vi "글로벌 1.vi"() -> ()   [LabVIEW 2017, in "Serial Communcation Devices Custom Device.lvlib"]
uses:
  Serial Communcation Devices Custom Device.lvlib
panel:
  in  "Channel Setting GUID":string
  out "GUID (Default Channel)":string="03D3BB99-1485-13A6-561D1F898F032919"
  in  "Flow Control":string
  in  "Stop Bits":string
  in  "Parity":string
  in  "Data Bits":string
  in  "Baud Rate":string
  in  "VISA Resource Name":string
  in  "Timeout(ms)":string
  in  "Enable Termination Char":string
  in  "Device GUID":string
  # "43b76903-71cc-4e2b-b034-344d1b7f9646"
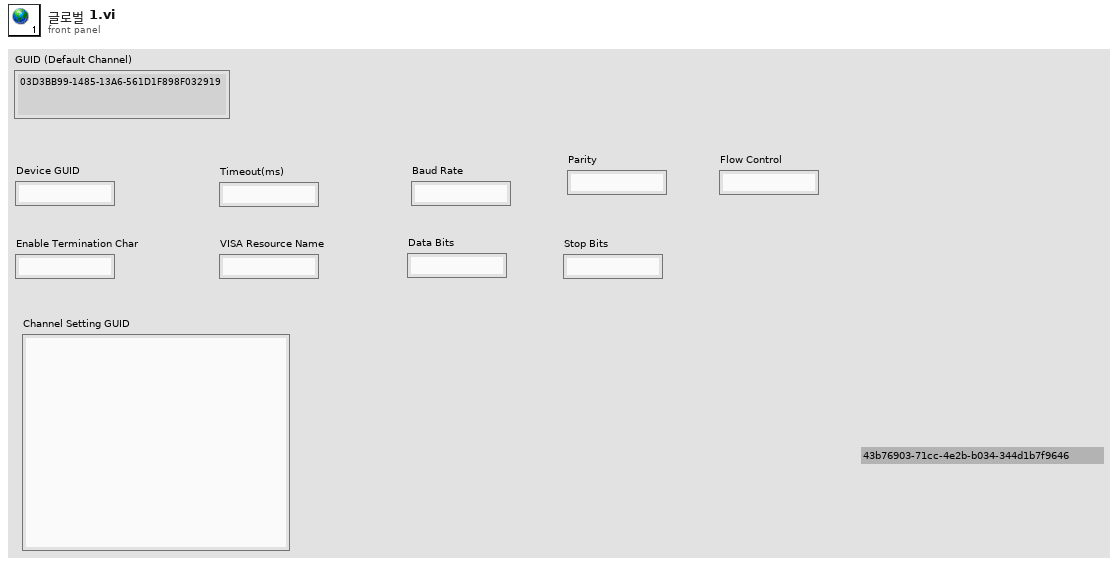
[diagram p1: front panel]
diagram:
